vi "get system information - example.vi"() -> ()   [LabVIEW 2014]
uses:
  classes/Controller/controller information.ctl
  classes/Controller/device information.ctl
  classes/Controller/network adapter settings.ctl
  classes/Chassis/chassis and module information.ctl
  classes/Chassis/chassis information.ctl
  classes/Module/module information.ctl
  classes/SysCfg Device/SysCfg Device.lvclass
  classes/Controller/Controller.lvclass
  classes/Chassis/Chassis.lvclass
  classes/Device/Device.lvclass
  classes/Module/Module.lvclass
panel:
  out "local chassis information":T1[](array[typedef]) {"chassis"."product ID" format="%.0x"; "modules"."product ID" format="%.0x"}
  in  "login":cluster{"User Name":string, "Password":string}={"User Name"="admin", "Password"=""}
  out "error out":errorcluster
  out "controller information":T4={"system session"=refnum, "system hardware ref"=refnum, "vendor name"="", "product name"="", "product ID"=0, "serial number"="", "device information"={"resource"="", "device class"="", "system start time"=timestamp(0 s since 1904-01-01), "current time"=timestamp(0 s since 1904-01-01), "time zone"="", "firmware revision"="", "image title"="", "image version"="", "system status"=""}, "primary network adapter"={"IP address"="", "MAC address"="", "IP address request mode"=1, "subnet mask"="", "gateway"="", "DNS server"="", "adapter mode"=1, "adapter type"=1}, "secondary network adapters"=[]} caption="Controller Information" {"product ID" format="%.0x"; "primary network adapter"."IP address request mode" items=["Static"=1, "DHCP/Link Local"=2, "Link-Local Only"=4, "DHCP Only"=8]; "primary network adapter"."adapter type" items=["Ethernet"=1, "WLAN"=2]; "primary network adapter"."adapter mode" items=["Disabled"=1, "TCP/IP Ethernet"=2, "Deterministic"=4, "EtherCAT"=8, "TCP/IP WLAN Connect"=32, "TCP/IP WLAN Create"=64]; "secondary network adapters"."IP address request mode" items=["Static"=1, "DHCP/Link Local"=2, "Link-Local Only"=4, "DHCP Only"=8]; "secondary network adapters"."adapter type" items=["Disabled"=1, "TCP/IP Ethernet"=2, "Deterministic"=4, "EtherCAT"=8, "TCP/IP WLAN Connect"=32, "TCP/IP WLAN Create"=64]; "secondary network adapters"."adapter mode" items=["Disabled"=1, "TCP/IP Ethernet"=2, "Deterministic"=4, "EtherCAT"=8, "TCP/IP WLAN Connect"=32, "TCP/IP WLAN Create"=64]}
  in  "target address (localhost)":string="localhost"
  # "NI Auth default settings \n(username: admin, \npassword: <blank>) are\nattempted automatically."
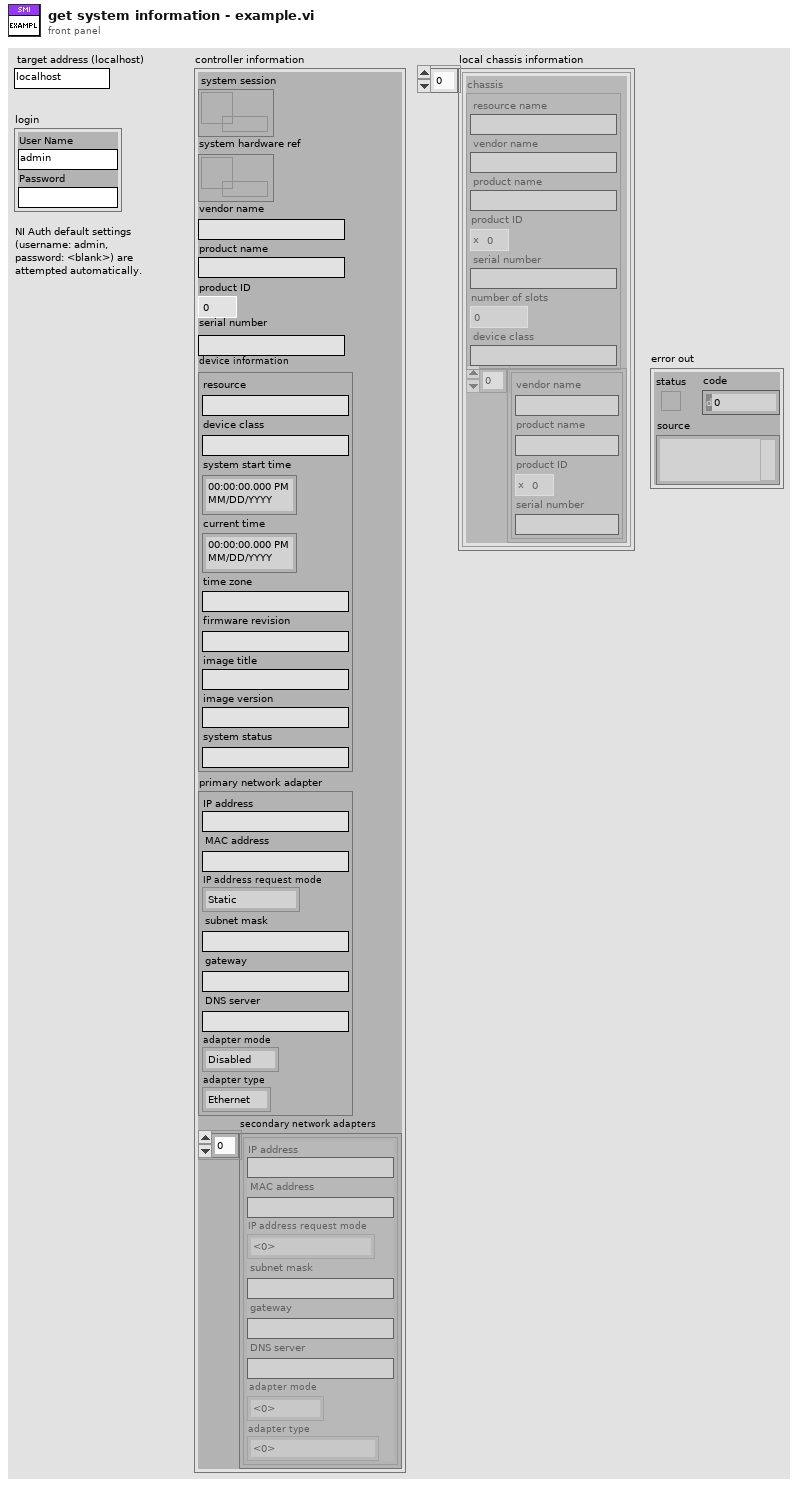
[diagram p1: front panel]
types:
  T1 = typedef "SMI.lvlib/Chassis.lvclass/chassis and module information.ctl" = cluster{"chassis":T2, "modules":T3[]}
  T2 = typedef "SMI.lvlib/Chassis.lvclass/chassis information.ctl" = cluster{"resource name":string, "vendor name":string, "product name":string, "product ID":u16, "serial number":string, "number of slots":i32, "device class":string}
  T3 = typedef "SMI.lvlib/Module.lvclass/module information.ctl" = cluster{"vendor name":string, "product name":string, "product ID":u16, "serial number":string}
  T4 = typedef "SMI.lvlib/Controller.lvclass/controller information.ctl" = cluster{"system session":refnum<data-value>, "system hardware ref":refnum<data-value>, "vendor name":string, "product name":string, "product ID":u16, "serial number":string, "device information":T5, "primary network adapter":T6, "secondary network adapters":T6[]}
  T5 = typedef "SMI.lvlib/Controller.lvclass/device information.ctl" = cluster{"resource":string, "device class":string, "system start time":timestamp, "current time":timestamp, "time zone":string, "firmware revision":string, "image title":string, "image version":string, "system status":string}
  T6 = typedef "SMI.lvlib/Controller.lvclass/network adapter settings.ctl" = cluster{"IP address":string, "MAC address":string, "IP address request mode":u32, "subnet mask":string, "gateway":string, "DNS server":string, "adapter mode":u32, "adapter type":u32}
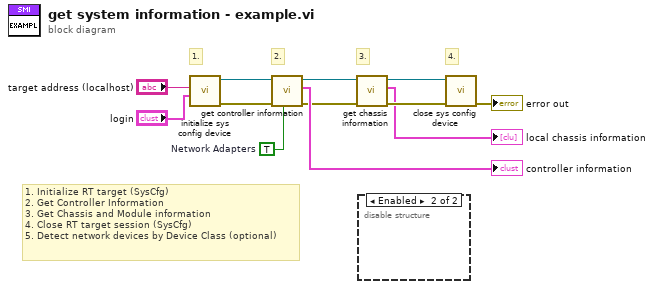
[diagram p0: block diagram]
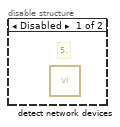
[diagram p2: hidden frame]
diagram:
  w6 = TRUE  # Network Adapters
  # "4."
  # "3."
  # "2."
  # "1."
  # "1. Initialize RT target (SysCfg)\n2. Get Controller Information\n3. Get Chassis and Module information\n4. Close RT target session (SysCfg)\n5. Detect network devices by Device Class (optional)"
  n1 = call "initialize sys config device.vi"("login"="login", "IP address (localhost)"="target address (localhost)") -> ("error out"=w7:errorcluster, "controller out"=w1:refnum<class "Controller.lvclass">)  [unwired: 8 in]
  n2 = call "get controller information.vi"("Network Adapters (F)"=w6, "error in"=w7, "controller in"=w1) -> ("error out"=w4:errorcluster, "controller information"=→"controller information":T4, "controller out"=w5:refnum<class "Controller.lvclass">)  [unwired: 6 in]
  n3 = call "get chassis information.vi"("error in"=w4, "controller in"=w5) -> ("error out"=w10:errorcluster, "local chassis"=→"local chassis information":T1[], "controller out"=w9:refnum<class "Controller.lvclass">)  [unwired: 6 in, 1 out]
  n4 = disable-structure shown="Enabled" {
    frame Disabled {
      # "5."
      n5 = call "detect network devices.vi"() -> ()  [unwired: 9 in, 3 out]
    }
    frame Enabled {
    }
  }
  n6 = call "close sys config device.vi"("error in"=w10, "controller in"=w9) -> ("error out"=→"error out":errorcluster)  [unwired: 8 in, 1 out]
